vi "MPX Get Path Names.vi"(8 "error in":errorcluster, 11 "session in":T1) -> (0 "error out":errorcluster, 2 "path tags":string[](array[string]), 3 "session out":T1)   [LabVIEW 2013]
doc: "Get path names for selected multiplexer."
uses:
  MPX Session.ctl
  MPX Type.ctl
  drivers/Multiplexers/Generic COM/GCOMM Session.ctl
  drivers/Multiplexers/Generic COM/GCOMM Signal.ctl
  drivers/Multiplexers/Generic COM/GCOMM Virtual Channel.ctl
  drivers/Multiplexers/Generic COM/GCOMM Logic State.ctl
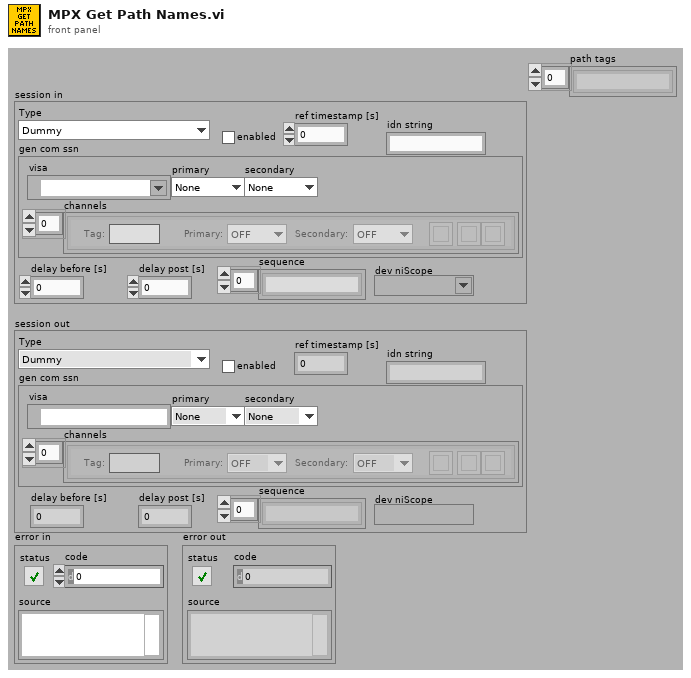
[diagram p1: front panel]
types:
  T1 = typedef "MPX Session.ctl" = cluster{"Type":T2, "gen com ssn":T3, "delay before [s]":dbl, "delay post [s]":dbl, "sequence":string[], "enabled":bool, "ref timestamp [s]":dbl, "idn string":string, "dev niScope":refnum<k15>}
  T2 = typedef "MPX Type.ctl" = enum16{"Dummy", "Generic - COM port", "Generic - niScope PFI"}
  T3 = typedef "GCOMM Session.ctl" = cluster{"visa":refnum<visa-resource-name>, "primary":T4, "secondary":T4, "channels":T5[]}
  T4 = typedef "GCOMM Signal.ctl" = enum16{"None", "DTR", "RTS"}
  T5 = typedef "GCOMM Virtual Channel.ctl" = cluster{"Primary:":T6, "Secondary:":T6, "btn clr":bool, "btn up":bool, "btn down":bool, "Tag:":string}
  T6 = typedef "GCOMM Logic State.ctl" = enum16{"OFF", "ON"}
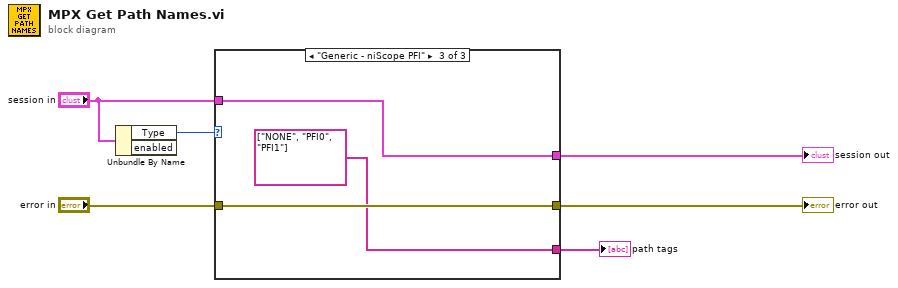
[diagram p0: block diagram]
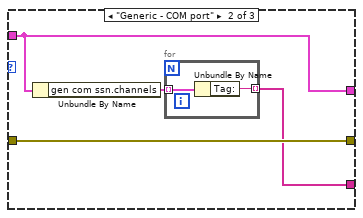
[diagram p3: hidden frame]
diagram:
  n1 = Unbundle By Name("session in") -> ("Type"=w6:T2)  [unwired: 1 out]
  n2 = case shown="\"Generic - niScope PFI\"" w6 {
    tunnel: "error in" -> [w7 w10 w16]
    tunnel: "session in" -> [w8 w12 w17]
    tunnel: [w8 w12 w17] -> w3
    tunnel: [w7 w10 w16] -> w2
    tunnel: [_ w9 string[] ["NONE", "PFI0", "PFI1"]] -> w1
    frame Default {
    }
    frame "Generic - COM port" {
      n3 = Unbundle By Name(w12) -> ("gen com ssn.channels"=w11:T5[])
      n4 = for {
        tunnel: w11 -> [w14] mode=indexing
        tunnel: [w13] -> w9 mode=indexing
        n5 = Unbundle By Name(w14) -> ("Tag:"=w13:string)
      }
    }
    frame "Generic - niScope PFI" {
    }
  }
  "error out" <- w2
  "session out" <- w3
  "path tags" <- w1
